vi "ThermalTune.vi"() -> ()   [LabVIEW 2016]
uses:
  <vilib>/Analysis/baseanly.llb/Mean (DBL).vi
  <vilib>/Utility/file.llb/Read Delimited Spreadsheet (DBL).vi
  <vilib>/gmath/NumericalOptimization/Nonlinear Curve Fit LM.vi
  <vilib>/gmath/NI_Gmath.lvlib
  <vilib>/Analysis/NI_AALBase.lvlib
panel:
  out "k (N/m)":dbl=0.8174 format="%#_3g"
  out "Geometric":dbl=0.8174 format="%_6e"
  out "Hutter (From Lorentzian Fit)":cluster{"A":dbl, "B":dbl, "P":dbl}={"A"=0.8174, "B"=0.8174, "P"=0.8174} {"P" format="%#_6e"; "B" format="%#_6e"; "A" format="%#_6e"}
  in  "Cantilever Parameters":T1={"kB (J/K)"=1.3806488e-23, "Pre-Factor"=0.8174, "Sensitivity(m/V)"=3.8e-08, "D (um)"=5.0, "L (um)"=42.0, "Phi (rad)"=0.2618, "T (K)"=297.0} {"Sensitivity(m/V)" format="%#_6p"; "Pre-Factor" format="%#_6e"; "kB (J/K)" format="%#_6e"}
  out "Parameter Guess":dbl[](array[numeric]) caption="pos\nwidth\namplitude*\noffset" format="%.4e"
  out "Best Fit Parameters":dbl[](array[numeric]) format="%.4e"
  out "XY Graph":cluster{cdb[]}[](graph)
  # "Instructions"
  # "Parameters of the Oscilloscope (From Graphs)"
  # "y = yo + [ H * (w/2)² / { (x - xc)²+(w/2)² } ]"
  # "yHutter = A / { (x - xc)²+B }"
  # "xc"
  # "w"
  # "H"
  # "P (area) = pi * A/ sqrt(B)"
  # "y0"
  # "Tip Height"
  # "Cantilever Length"
  # "Angle"
  # "k=Geometric*Prefactor * kB*T/(sensitivity^2*P)"
  # "Close Excitation window if open. Switch to contact mode.\nRemove High pass filter on AI0, connect Vert Deflection."
  # "Take a Ramp for sensitivity. Record a nice Tune with the oscilloscope.\nSave the PSD by clicking on the Save button with k enabled Icon"
  # "1us"
  # "40000"
  # "PSD zoom"
  # "Center = Center of the thermal Peak"
  # "Span = 30-50kHz"
  # "Resolution = 1Hz"
  # "Sampling = 1MS"
  # "PS Density\nHanning"
  # "RMS Averaging\nrms    V2"
  # "Exponential\n50ohm   one"
  # "3000"
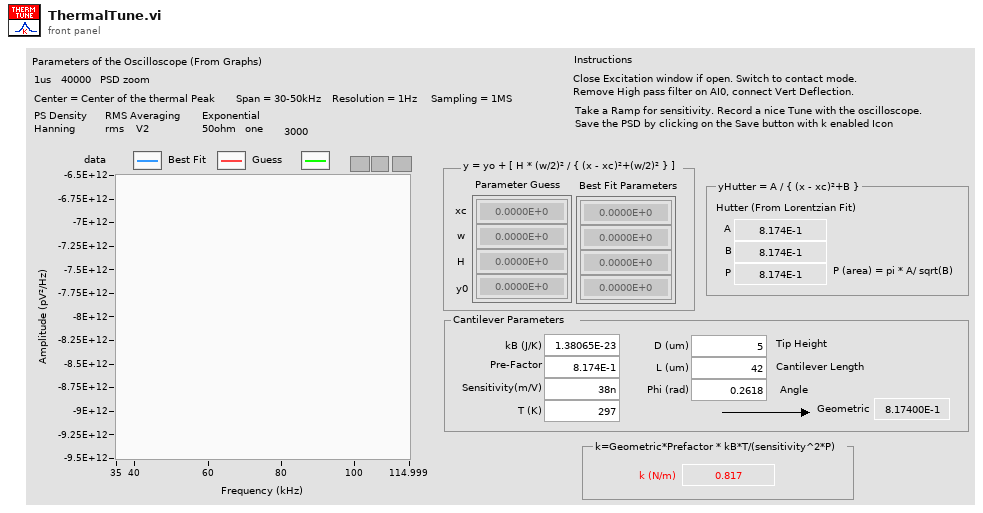
[diagram p1: front panel]
types:
  T1 = cluster{"kB (J/K)":dbl, "Pre-Factor":dbl, "Sensitivity(m/V)":dbl, "D (um)":dbl, "L (um)":dbl, "Phi (rad)":dbl, "T (K)":dbl}
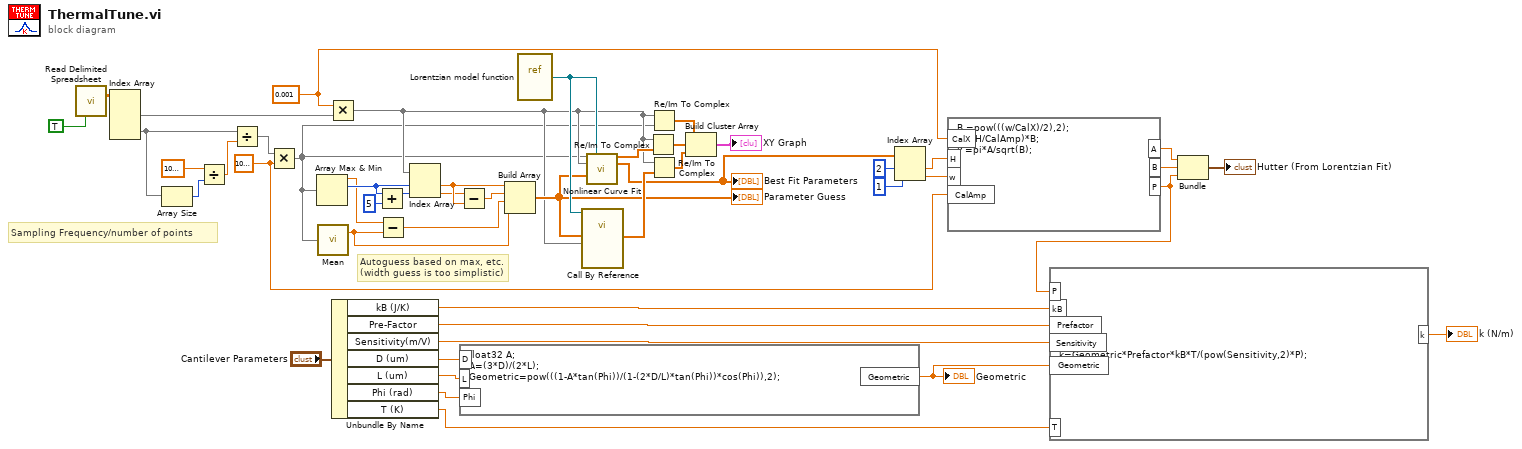
[diagram p0: block diagram]
diagram:
  w8 = 1000000000000.0
  w9 = 0.001
  # "Sampling Frequency/number of points"
  # "Autoguess based on max, etc.\n(width guess is too simplistic)"
  n1 = call-poly <vilib>:"Read Delimited Spreadsheet.vi"("transpose? (F)"=TRUE) -> ("all rows"=w47:dbl[][])  [unwired: 9 in, 5 out]
  n2 = Index Array(array=w47) -> (element #1=w37:dbl[], element #2=w3:dbl[])  [unwired: 4 in]
  n3 = Array Size(array=w3) -> (size(s)=w4:i32)
  n4 = Divide(x=1000000.0, y=w4) -> (x/y=w5:dbl)
  n5 = Divide(x=w3, y=w5) -> (x/y=w7:dbl[])
  n6 = Multiply(x=w7, y=w8) -> (x*y=w29:dbl[])
  n7 = Array Max & Min(array=w29) -> (max value=w33:dbl, max index (indices)=w45:i32)  [unwired: 2 out]
  n8 = call-poly <vilib>:"Mean.vi"("X"=w29) -> ("mean"=w34:dbl)  [unwired: 1 out]
  n9 = Multiply(x=w9, y=w37) -> (x*y=w30:dbl[])
  n10 = Unbundle By Name("Cantilever Parameters") -> ("kB (J/K)"=w19:dbl, "Pre-Factor"=w18:dbl, "Sensitivity(m/V)"=w17:dbl, "D (um)"=w15:dbl, "L (um)"=w14:dbl, "Phi (rad)"=w13:dbl, "T (K)"=w12:dbl)
  n11 = Add(x=w45, y=5) -> (x+y=w44:i32)
  n12 = Subtract(x=w33, y=w34) -> (x-y=w31:dbl)
  n13 = Index Array(array=w30, index #1=w45, index #2=w44) -> (element #1=w42:dbl, element #2=w41:dbl)
  n14 = Subtract(x=w41, y=w42) -> (x-y=w39:dbl)
  n15 = formula code="float32 A;\nA=(3*D)/(2*L);\nGeometric=pow(((1-A*tan(Phi))/(1-(2*D/L)*tan(Phi))*cos(Phi)),2);"("D"=w15, "L"=w14, "Phi"=w13) -> ("Geometric"=w11:dbl)
  "Geometric" <- w11
  n16 = Build Array(w42, w39, w31, w34) -> (w32:dbl[])
  "Parameter Guess" <- w32
  n17 = vi-ref "Lorentzian model function.vi"() -> (w38:refnum<vi>)
  n18 = call-by-ref "?"(reference=w38, "X"=w30, "a"=w32) -> ("f(X,a)"=w36:dbl[])  [unwired: 3 in, 4 out]
  n19 = call-poly <vilib>:"Nonlinear Curve Fit.vi"("Y"=w29, "f(x,a)"=w38, "X"=w30, "initial parameters"=w32) -> ("best nonlinear fit"=w35:dbl[], "best fit parameters"=w28:dbl[])  [unwired: 6 in, 4 out]
  "Best Fit Parameters" <- w28
  n20 = Re/Im To Complex(1:w35, 2:w30) -> (0:w1:cdb[])
  n21 = Re/Im To Complex(1:w29, 2:w30) -> (0:w46:cdb[])
  n22 = Re/Im To Complex(1:w36, 2:w30) -> (0:w2:cdb[])
  n23 = Build Cluster Array(w46, w1, w2) -> (→"XY Graph":cluster{cdb[]}[])
  n24 = Index Array(array=w28, index #1=2 ("index"), index #2=1 ("index")) -> (element #1=w25:dbl, element #2=w24:dbl)
  n25 = formula code="B =pow(((w/CalX)/2),2);\nA=(H/CalAmp)*B;\nP =pi*A/sqrt(B);"("H"=w25, "w"=w24, "CalAmp"=w8, "CalX"=w9) -> ("A"=w23:dbl, "B"=w22:dbl, "P"=w16:dbl)
  n26 = formula code="k=Geometric*Prefactor*kB*T/(pow(Sensitivity,2)*P);"("kB"=w19, "Prefactor"=w18, "Sensitivity"=w17, "Geometric"=w11, "P"=w16, "T"=w12) -> ("k"=→"k (N/m)":dbl)
  n27 = Bundle("A"=w23, "B"=w22, "P"=w16) -> (→"Hutter (From Lorentzian Fit)":cluster{"A":dbl, "B":dbl, "P":dbl})  [unwired: 1 in]
